vi "Agilent E363X Series Output DC Volts - OVP OCP.vi"() -> ()   [LabVIEW 2010]
doc: "This example shows how to configure the instrument's output voltage level, over current protection, and over voltage protection. The actual voltage level and actual current level are returned as well as status of OVP or OCP being tripped.\n\n<B>Note:</B> The E3631 does not support over voltage protection or the seletion of voltage range. This example does not support the E3631."
uses:
  <instrlib>/Agilent E363X Series/Agilent E363X Series.lvlib
panel:
  in  "Current Limit (0.0 A)":dbl=1.0 format="%.3g"
  in  "Behavior (0: Regulate)":u16(ring) items=["Regulate", "Trip"]
  in  "Voltage Limit (0.0 V)":dbl=5.0 format="%.3g"
  out "Actual Current Level (A)":dbl format="%.3g"
  out "Actual Voltage Level (V)":dbl format="%.3g"
  in  "Voltage Level (0.0 V)":dbl=1.0 format="%.3g"
  in  "Enable OVP (T: Enable)":bool=TRUE
  in  "Voltage Range (0: Low)":u16(ring) items=["Low", "High"]
  in  "Stop Output":bool
  out "OCP Tripped?":bool
  out "OVP Tripped?":bool
  in  "VISA resource name":refnum<visa-resource-name>
  # "(c) 2008 National Instruments.  ALL RIGHTS RESERVED."
  # "Voltage Settings"
  # "Note: The E3631 does not support over voltage protection or the selection of voltage range. This example does not support the E3631."
  # "Over Voltage Protection"
  # "Over Current Protection"
  # "Measurements"
  # "OVP/OCP Status"
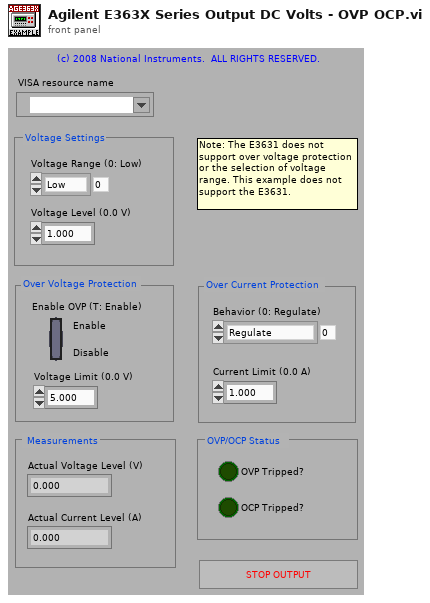
[diagram p1: front panel]
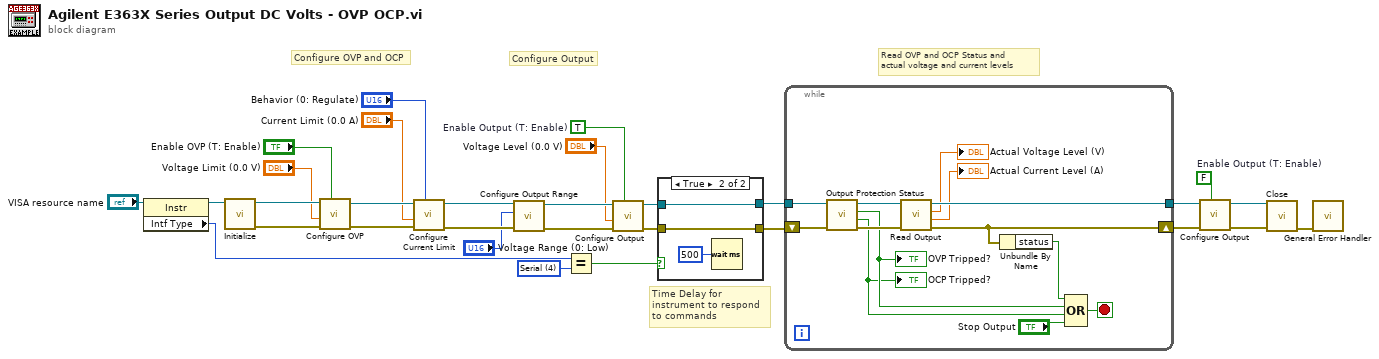
[diagram p0: block diagram]
diagram:
  w3 = u16 4 items=["GPIB"=1, "VXI"=2, "GPIB-VXI"=3, "Serial"=4, "PXI"=5, "TCPIP"=6, "USB"=7] ("Interface Information:Interface Type")
  w18 = TRUE  # Enable Output (T: Enable)
  w25 = FALSE  # Enable Output (T: Enable)
  # "Time Delay for instrument to respond to commands"
  # "Read OVP and OCP Status and\nactual voltage and current levels"
  # "Configure Output"
  # "Configure OVP and OCP"
  n1 = property class="Instr"(reference="VISA resource name") -> (reference out=w5:refnum<visa-resource-name>, "Intf Type"=w2:u16)  [unwired: 1 in, 1 out]
  n2 = call <instrlib>:"Initialize.vi"("VISA resource name"=w5) -> ("error out"=w28:errorcluster, "VISA resource name out"=w29:refnum<visa-resource-name>)  [unwired: 9 in]
  n3 = call <instrlib>:"Configure OVP.vi"("Enable OVP (T: Enable)"="Enable OVP (T: Enable)", "error in (no error)"=w28, "Voltage Limit (0.0 V)"="Voltage Limit (0.0 V)", "VISA resource name"=w29) -> ("error out"=w27:errorcluster, "VISA resource name out"=w26:refnum<visa-resource-name>)  [unwired: 6 in]
  n4 = call <instrlib>:"Configure Current Limit.vi"("Behavior (0: Regulate)"="Behavior (0: Regulate)", "error in (no error)"=w27, "Current Limit (0.0 A)"="Current Limit (0.0 A)", "VISA resource name"=w26) -> ("error out"=w16:errorcluster, "VISA resource name out"=w17:refnum<visa-resource-name>)  [unwired: 6 in]
  n5 = call <instrlib>:"Configure Output Range.vi"("error in (no error)"=w16, "Voltage Range (0: Low)"="Voltage Range (0: Low)", "VISA resource name"=w17) -> ("error out"=w19:errorcluster, "VISA resource name out"=w20:refnum<visa-resource-name>)  [unwired: 7 in]
  n6 = Equal?(x=w2, y=w3) -> (x = y?=w1:bool)
  n7 = call <instrlib>:"Configure Output.vi"("Enable Output (T: Enable)"=w18, "error in (no error)"=w19, "Voltage Level (0.0 V)"="Voltage Level (0.0 V)", "VISA resource name"=w20) -> ("error out"=w6:errorcluster, "VISA resource name out"=w9:refnum<visa-resource-name>)  [unwired: 6 in]
  n8 = case shown="True" w1 {
    tunnel: [w32 w34] -> w8
    tunnel: w9 -> [w32 w34]
    tunnel: [w31 w33] -> w7
    tunnel: w6 -> [w31 w33]
    frame False {
    }
    frame True {
      n9 = Wait (ms)(milliseconds to wait=u32 500) -> ()  [unwired: 1 out]
    }
  }
  n10 = while {
    tunnel: w8 -> [w42]
    tunnel: [w48] -> w21
    shift-right: [w44] -> w23
    shift-left: w7 -> [w41]
    stop <- w45 stop-if-true
    n11 = call <instrlib>:"Output Protection Status.vi"("error in (no error)"=w41, "VISA resource name"=w42) -> ("error out"=w46:errorcluster, "OCP Tripped?"=w37:bool, "OVP Tripped?"=w38:bool, "VISA resource name out"=w47:refnum<visa-resource-name>)  [unwired: 6 in]
    "OVP Tripped?" <- w38
    "OCP Tripped?" <- w37
    n12 = call <instrlib>:"Read Output.vi"("error in (no error)"=w46, "VISA resource name"=w47) -> ("error out"=w44:errorcluster, "Actual Current Level (A)"=→"Actual Current Level (A)":dbl, "Actual Voltage Level (V)"=→"Actual Voltage Level (V)":dbl, "VISA resource name out"=w48:refnum<visa-resource-name>)  [unwired: 6 in]
    n13 = Unbundle By Name(w44) -> ("status"=w43:bool)
    n14 = Compound Arithmetic op=OR(w43, w38, w37, "Stop Output") -> (w45:bool)
  }
  n15 = call <instrlib>:"Configure Output.vi"("Enable Output (T: Enable)"=w25, "error in (no error)"=w23, "VISA resource name"=w21) -> ("error out"=w22:errorcluster, "VISA resource name out"=w24:refnum<visa-resource-name>)  [unwired: 7 in]
  n16 = call <instrlib>:"Close.vi"("error in (no error)"=w22, "VISA resource name"=w24) -> ("error out"=w30:errorcluster)  [unwired: 9 in]
  n17 = call <vilib>:"General Error Handler.vi"("error in (no error)"=w30) -> ()  [unwired: 10 in, 5 out]
